vi "JoystickNetworkTableHandler.vi"(0 "JoystickDevRef":T1) -> ()   [LabVIEW 2012]
uses:
  <vilib>/Rock Robotics/WPI/Joystick/WPI_JoystickDevRef.ctl
  <vilib>/Rock Robotics/WPI/Joystick/WPI_JoystickDeviceEnum.ctl
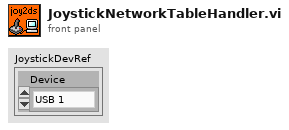
[diagram p1: front panel]
types:
  T1 = typedef "WPI_JoystickDevRef.ctl" = cluster{"Device":T2}
  T2 = typedef "WPI_JoystickDeviceEnum.ctl" = enum16{"USB 1", "USB 2", "USB 3", "USB 4", "Kinect 1", "Kinect 2"}
  T3 = typedef "WPI_JoystickButtonState.ctl" = cluster{"Button 1":bool, "Button 2":bool, "Button 3":bool, "Button 4":bool, "Button 5":bool, "Button 6":bool, "Button 7":bool, "Button 8":bool, "Button 9":bool, "Button 10":bool, "Button 11":bool, "Button 12":bool}
  T4 = cluster{"axis 1 (x)":dbl, "axis 2 (y)":dbl, "axis 3 (throttle)":dbl, "axis 4":dbl, "axis 5":dbl, "axis 6":dbl}
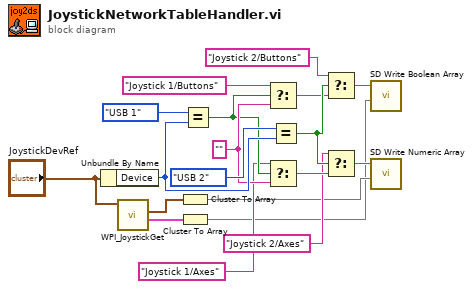
[diagram p0: block diagram]
diagram:
  w10 = "" ("f")
  n1 = Unbundle By Name("JoystickDevRef") -> ("Device"=w11:T2)
  n2 = call <vilib>:"WPI_JoystickGet.vi"("JoystickDevRef"="JoystickDevRef") -> ("Buttons"=w4:T3, "Axes"=w3:T4)  [unwired: 1 in, 4 out]
  n3 = Cluster To Array(cluster=w3) -> (array=w6:dbl[])
  n4 = Cluster To Array(cluster=w4) -> (array=w5:bool[])
  n5 = Equal?(x=WPI_JoystickDeviceEnum."USB 1", y=w11) -> (x = y?=w9:bool)
  n6 = Select(t="Joystick 1/Buttons" ("Name"), s=w9, f=w10) -> (s? t:f=w15:string)
  n7 = Select(t="Joystick 1/Axes" ("Name"), s=w9, f=w10) -> (s? t:f=w16:string)
  n8 = Equal?(x=WPI_JoystickDeviceEnum."USB 2", y=w11) -> (x = y?=w19:bool)
  n9 = Select(t="Joystick 2/Buttons" ("Name"), s=w19, f=w15) -> (s? t:f=w18:string)
  n10 = Select(t="Joystick 2/Axes" ("Name"), s=w19, f=w16) -> (s? t:f=w17:string)
  n11 = call <vilib>:"SD Write Boolean Array.vi"("Boolean Array"=w5, "Name"=w18) -> ()  [unwired: 8 in, 2 out]
  n12 = call <vilib>:"SD Write Numeric Array.vi"("Numeric Array"=w6, "Name"=w17) -> ()  [unwired: 8 in, 2 out]
